vi "subvi_read_metadata.vi"(1 "Pfad":path) -> (0 "Metadata":T1)   [LabVIEW 2016]
uses:
  cluster_metadata.ctl
  <vilib>/Utility/file.llb/Read Delimited Spreadsheet (string).vi
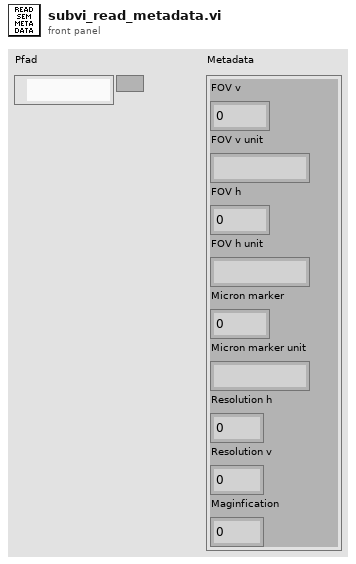
[diagram p1: front panel]
types:
  T1 = typedef "cluster_metadata.ctl" = cluster{"FOV v":dbl, "FOV v unit":string, "FOV h":dbl, "FOV h unit":string, "Micron marker":dbl, "Micron marker unit":string, "Resolution h":i32, "Resolution v":i32, "Maginfication":i32}
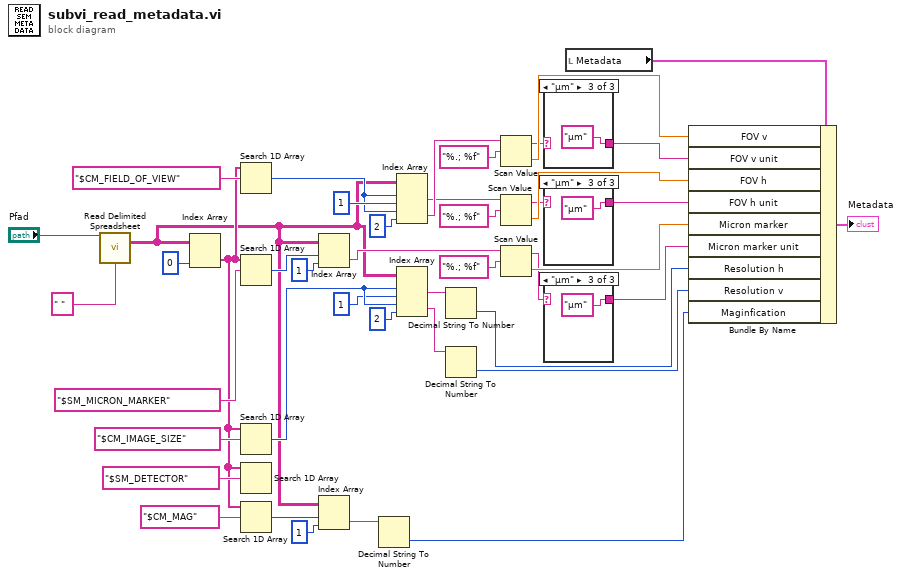
[diagram p0: block diagram]
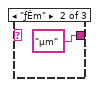
[diagram p3: hidden frame]
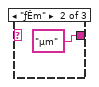
[diagram p5: hidden frame]
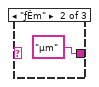
[diagram p7: hidden frame]
diagram:
  n1 = call-poly <vilib>:"Read Delimited Spreadsheet.vi"("file path (dialog if empty)"="Pfad", "delimiter (\\t)"=" " ("delimiter (\\t)")) -> ("all rows"=w19:string[][])  [unwired: 8 in, 5 out]
  n2 = Index Array(array=w19, index (col)=0 ("Deaktivierter Index (Spalte)")) -> (element=w28:string[])  [unwired: 1 in]
  n3 = Search 1D Array(1D array=w28, element="$CM_FIELD_OF_VIEW" ("Element")) -> (index of element=w35:i32)  [unwired: 1 in]
  n4 = Search 1D Array(1D array=w28, element="$SM_MICRON_MARKER" ("Element")) -> (index of element=w27:i32)  [unwired: 1 in]
  n5 = Search 1D Array(1D array=w28, element="$CM_IMAGE_SIZE" ("Element")) -> (index of element=w24:i32)  [unwired: 1 in]
  n6 = Search 1D Array(1D array=w28, element="$SM_DETECTOR" ("Element")) -> ()  [unwired: 1 in, 1 out]
  n7 = Search 1D Array(1D array=w28, element="$CM_MAG" ("Element")) -> (index of element=w18:i32)  [unwired: 1 in]
  n8 = Index Array(array=w19, index (row)=w27, index (col)=1 ("Deaktivierter Index (Spalte)")) -> (element=w25:string)
  n9 = Index Array(array=w19, index (row)=w18, index (col)=1 ("Deaktivierter Index (Spalte)")) -> (element=w16:string)
  n10 = Decimal String To Number(string=w16) -> (number=w9:i32)  [unwired: 2 in, 1 out]
  n11 = Index Array(array=w19, index (row) #1=w35, index (col) #1=1 ("Deaktivierter Index (Spalte)"), index (row) #2=w35, index (col) #2=2 ("Deaktivierter Index (Spalte)")) -> (element #1=w30:string, element #2=w32:string)
  n12 = Index Array(array=w19, index (row) #1=w24, index (col) #1=1 ("Deaktivierter Index (Spalte)"), index (row) #2=w24, index (col) #2=2 ("Deaktivierter Index (Spalte)")) -> (element #1=w21:string, element #2=w20:string)
  n13 = Decimal String To Number(string=w21) -> (number=w11:i32)  [unwired: 2 in, 1 out]
  n14 = Decimal String To Number(string=w20) -> (number=w10:i32)  [unwired: 2 in, 1 out]
  n15 = Scan Value(string=w32, format string="%.; %f" ("Format-String")) -> (output string=w7:string, value=w13:dbl)  [unwired: 1 in]
  n16 = Scan Value(string=w30, format string="%.; %f" ("Format-String")) -> (output string=w4:string, value=w8:dbl)  [unwired: 1 in]
  n17 = Scan Value(string=w25, format string="%.; %f" ("Format-String")) -> (output string=w2:string, value=w12:dbl)  [unwired: 1 in]
  n18 = case shown="\"µm\"" w7 {
    selector: w7 -> [w44 _ _]
    tunnel: [w44 "µm" "µm"] -> w6
    frame "encoding ok", Default {
    }
    frame "ƒÊm" {
    }
    frame "µm" {
    }
  }
  n19 = case shown="\"µm\"" w4 {
    selector: w4 -> [w47 _ _]
    tunnel: [w47 "µm" "µm"] -> w3
    frame "encoding ok", Default {
    }
    frame "ƒÊm" {
    }
    frame "µm" {
    }
  }
  n20 = case shown="\"µm\"" w2 {
    selector: w2 -> [w50 _ _]
    tunnel: [w50 "µm" "µm"] -> w1
    frame "encoding ok", Default {
    }
    frame "ƒÊm" {
    }
    frame "µm" {
    }
  }
  n21 = local read "Metadata"() -> (w14:T1)
  n22 = Bundle By Name(cluster=w14, "FOV v"=w13, "FOV v unit"=w6, "FOV h"=w8, "FOV h unit"=w3, "Micron marker"=w12, "Micron marker unit"=w1, "Resolution h"=w11, "Resolution v"=w10, "Maginfication"=w9) -> (→"Metadata":T1)
